vi "clear Session Data.vi"(0 "OBJ - Measurement Session in":refnum<class "FPGA Session.lvclass">, 11 "error in":errorcluster) -> (4 "OBJ - Measurement Session out":refnum<class "FPGA Session.lvclass">, 15 "error out":errorcluster)   [LabVIEW 2015, in "FPGA Session.lvclass"]
doc: "OVERRIDE VI\nPlaceholder for decendant classes to clear session information and close references."
uses:
  FPGA Session.lvclass
  FPGA Session.lvclass/FPGA Session.ctl
  <vilib>/FPGAPlugInAG/cRIO-9081/niLvFpga_Close_cRIO-9081.vi
  <vilib>/rvi/errors/niLvFpgaAdjustHostInterfaceError.vi
  <vilib>/Utility/error.llb/Error Cluster From Error Code.vi
  <vilib>/rvi/interface/nirviCloseFPGA/nirviCloseFPGA.xnode
  FPGA Ref.ctl
  FPGA Bitfiles/Nicholas.lvbitx
  <vilib>/rvi/interface/nirviReadWriteControl/nirviReadWriteControl.xnode
  NiFpgaLv.dll
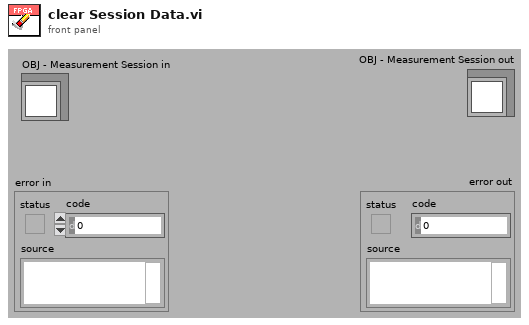
[diagram p1: front panel]
types:
  T1 = typedef "FPGA Ref.ctl" = refnum<k20>
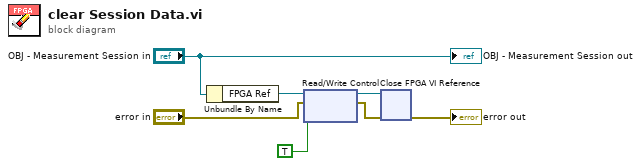
[diagram p0: block diagram]
diagram:
  n1 = Unbundle By Name("OBJ - Measurement Session in") -> ("FPGA Ref"=w4:T1)
  n2 = xnode "Read/Write Control"("FPGA VI Reference In"=w4, "error in"="error in", "Stop"=TRUE) -> ("FPGA VI Reference Out"=w3:T1, "error out"=w1:errorcluster)
  n3 = xnode "Close FPGA VI Reference"("FPGA VI Reference In"=w3, "error in"=w1) -> ("error out"=→"error out":errorcluster)
  "OBJ - Measurement Session out" <- "OBJ - Measurement Session in"
